vi "Test Add Sheet.vi"(11 "Test Case In":refnum<class "Test Open Xml.lvclass">) -> (0 "error out":errorcluster, 3 "Test Case Out":refnum<class "Test Open Xml.lvclass">)   [LabVIEW 2020, in "Test Open Xml.lvclass"]
uses:
  Test Open Xml.lvclass
  Source/Open Xml.lvlib
  3fd9ecb3-cb99-4db2-8a80-5e80f6af10ae.vi
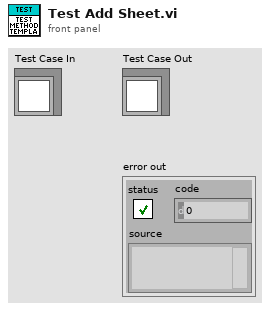
[diagram p1: front panel]
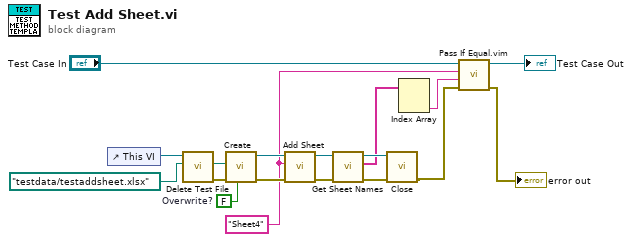
[diagram p0: block diagram]
diagram:
  w1 = FALSE  # Overwrite?
  w7 = "Sheet4" ("SheetName")
  n1 = control-ref of="This VI"() -> (w4:refnum<vi>)
  n2 = call "Delete Test File.vi"("name or relative path"=path "testdata/testaddsheet.xlsx", "VI in"=w4) -> ("error out"=w3:errorcluster, "deleted path"=w2:path)  [unwired: 8 in]
  n3 = call "Create.vi"("Overwrite?"=w1, "error in"=w3, "Path"=w2) -> ("error out"=w15:errorcluster, "SpreadsheetDoc"=w13:refnum<k24>)  [unwired: 7 in]
  n4 = call "Add Sheet.vi"("error in"=w15, "Sheet Name"=w7, "SpreadsheetDoc in"=w13) -> ("error out"=w14:errorcluster, "SpreadsheetDoc out"=w10:refnum<k24>)  [unwired: 7 in]
  n5 = call "Get Sheet Names.vi"("error in"=w14, "SpreadsheetDoc in"=w10) -> ("error out"=w11:errorcluster, "Sheet Names"=w8:string[], "SpreadsheetDoc out"=w9:refnum<k24>)  [unwired: 7 in]
  n6 = call "Close.vi"("error in"=w11, "SpreadsheetDoc"=w9) -> ("error out"=w12:errorcluster)  [unwired: 9 in]
  n7 = Index Array(array=w8) -> (element #2=w6:string)  [unwired: 2 in, 1 out]
  n8 = call "Pass If Equal.vim"("error in (no error)"=w12, "Actual"=w6, "Expected"=w7, "LUnit Test Case In"="Test Case In") -> ("error out"=→"error out":errorcluster, "LUnit Test Case Out"=→"Test Case Out":refnum<class "Test Open Xml.lvclass">)  [unwired: 6 in]
